vi "Write VISA address.vi"(8 "error in (no error)":errorcluster, 10 "VISA address":refnum<visa-resource-name>="GPIB0::22::INSTR", 11 "PS Driver in":refnum<class "PS Driver.lvclass">) -> (0 "error out":errorcluster, 3 "PS Driver out":refnum<class "PS Driver.lvclass">)   [LabVIEW 2019, in "PS Driver.lvlib" / "PS Driver.lvclass"]
uses:
  PS Driver.lvclass
  PS Driver.lvclass/PS Driver.ctl
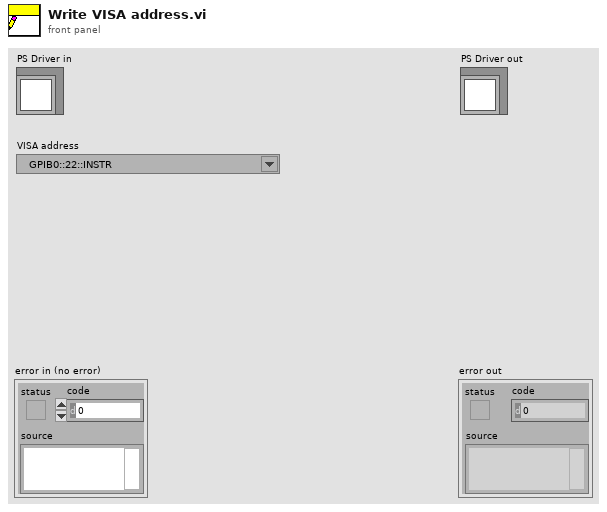
[diagram p1: front panel]
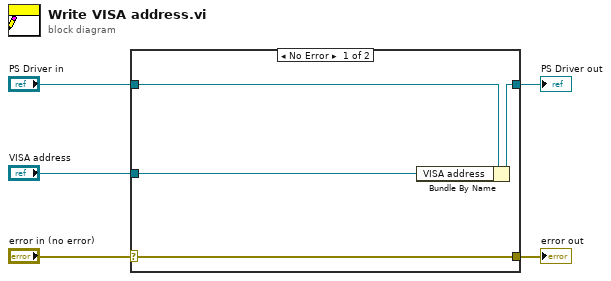
[diagram p0: block diagram]
diagram:
  n1 = case shown="No Error" "error in (no error)" {
    selector: "error in (no error)" -> [w9 w10]
    tunnel: [w9 w10] -> w4
    tunnel: [w7 w11] -> w2
    tunnel: "PS Driver in" -> [w8 w11]
    tunnel: "VISA address" -> [w6 _]
    frame No Error {
      n2 = Bundle By Name(cluster=w8, "VISA address"=w6) -> (w7:refnum<class "PS Driver.lvclass">)
    }
    frame Error {
    }
  }
  "error out" <- w4
  "PS Driver out" <- w2
